vi "Simple.vi"() -> ()   [LabVIEW 2019]
doc: "A simple demonstration of encoding a cluster as MessagePack data and then decoding the MessagePack data back into the cluster. This shows how to use the high-level To Msgpack and From Msgpack VIs to convert anything into MessagePack data and convert MessagePack data based on a schema."
uses:
  vi.lib/Field R&D Services/LabPack/LabPack.lvlib
panel:
  in  "Input":cluster{"Compact":bool, "Schema":i32}={"Compact"=TRUE, "Schema"=0}
  out "Msgpack Data":string
  out "Output":cluster{"Compact":bool, "Schema":i32}
  # "Run the VI to see the input cluster encoded as MessagePack data and then decoded back to a cluster."
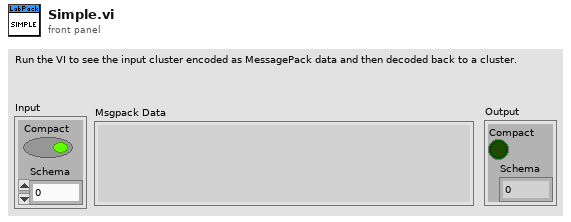
[diagram p1: front panel]
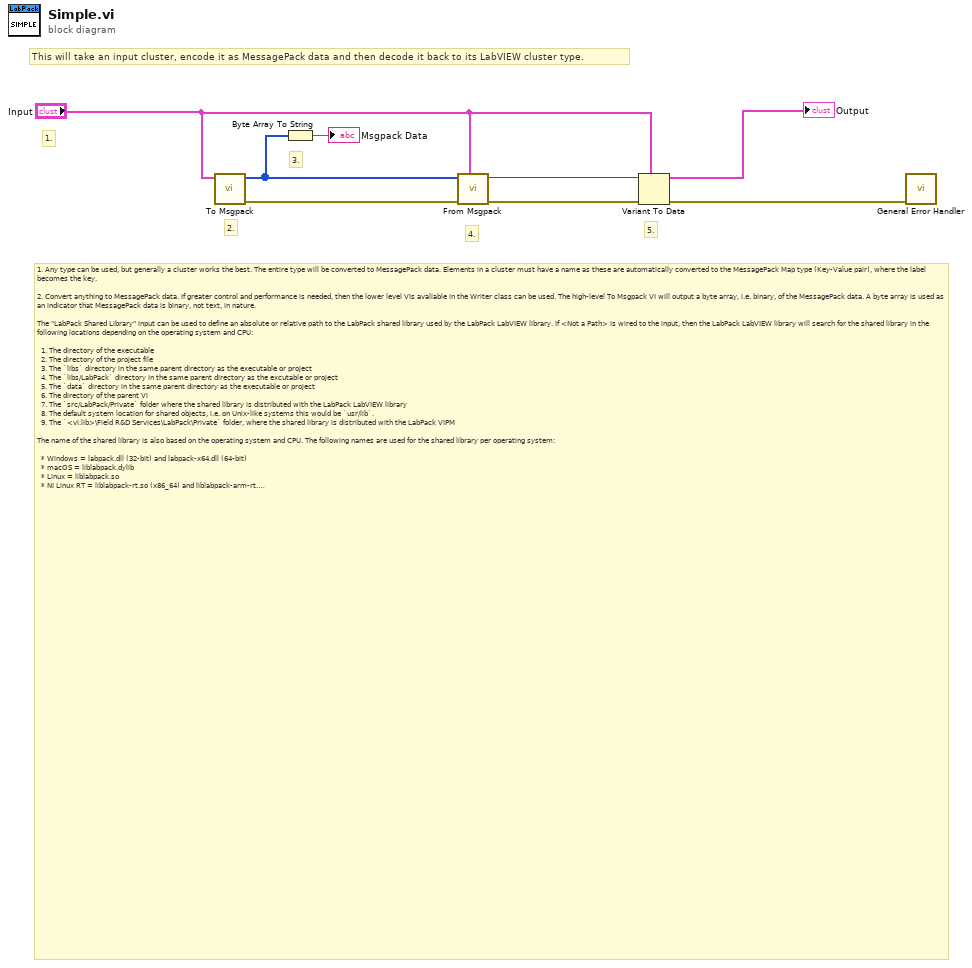
[diagram p0: block diagram]
diagram:
  # "1."
  # "This will take an input cluster, encode it as MessagePack data and then decode it back to its LabVIEW cluster type."
  # "1. Any type can be used, but generally a cluster works the best. The entire type will be converted to MessagePack data. Elements in a cluster must have a name as these are automatically converted to the MessagePack Map type (Key-Value pair), where the label becomes the key.\n\n2. Convert anything to MessagePack data. If greater control and performance is needed, then the lower level VIs avaliable in the Writer class can be used. The high-level To Msgpack VI will output a byte array, i.e. binary, of the MessagePack data. A byte array is used as an indicator that MessagePack data is binary, not text, in nature. \n\nThe \"LabPack Shared Library\" input can be used to define an absolute or relative path to the LabPack shared library used by the LabPack LabVIEW library. If <Not a Path> is wired to the input, then the LabPack LabVIEW library will search for the shared library in the following locations depending on the operating system and CPU: \n\n  1. The directory of the executable \n  2. The directory of the project file\n  3. The `libs` directory in the same parent directory as the executable or project\n  4. The `libs/LabPack` directory in the same parent directory as the excutable or project\n  5. The `data` directory in the same parent directory as the executable or project\n  6. The directory of the parent VI\n  7. The `src/LabPack/Private` folder where the shared library is distributed with the LabPack LabVIEW library\n  8. The default system location for shared objects, i.e. on Unix-like systems this would be `usr/lib`.\n  9. The `<vi.lib>\\Field R&D Services\\LabPack\\Private` folder, where the shared library is distributed with the LabPack VIPM\n\nThe name of the shared library is also based on the operating system and CPU. The following names are used for the shared library per operating system:\n\n  * Windows = labpack.dll (32-bit) and labpack-x64.dll (64-bit)\n  * macOS = liblabpack.dylib\n  * Linux = liblabpack.so\n  * NI Linux RT = liblabpack-rt.so (x86_64) and liblabpack-arm-rt.so (ARM)\n\nIf building a real-time application or executable with the Application Builder, the appropriate shared library must be installed on the target machine. For example, the liblabpack-rt.so must be transferred and \"installed\" on a NI Linux RT remote target in one of the locations listed above or in another location with a known path that can be passed to the \"LabPack Shared Library\" input.\n\n(i) Current Working Directory, (ii) the source (src) folder, and the system-specific shared library folder, i.e. \"/usr/lib/\" on Unix-like operating systems including Real-Time targets. The LabPack shared library must be present on disk. When creating an executable that uses the LabPack library, ensure the LabPack shared library is installed on the target in a known location and this path is used with the \"LabPack Shared Library\" input.\n\n3. Use the Byte Array to String primitive to make the MessagePack data more human-readable as a string in hex notation. Note, MessagePack data is binary and thus best viewed by a human in hex notation.\n\n4. Convert a byte array, i.e. binary data, in the MessagePack format to a LabVIEW type based on a \"schema\", which indicates the structure of the MessagePack data. Currently, the LabPack library does NOT support schema-less decoding of MessagePack data. If greater control and/or performance is needed, then the lower level VIs available in the Reader class can be used. The high-level From Msgpack VI is essentially a wrapper for the low-level Reader VIs. The \"LabPack Shared Library\" input can be used to define an absolute path to the LabPack shared library used by the LabPack LabVIEW library. If Not a Path is wired to the input, then the LabPack LabVIEW library will search for the shared library in the following locations: (i) Current Working Directory, (ii) the source (src) folder, and the system-specific shared library folder, i.e. \"/usr/lib/\" on Unix-like operating systems including Real-Time targets. The LabPack shared library must be present on disk. When creating an executable that uses the LabPack library, ensure the LabPack shared library is installed on the target in a known location and this path is used with the \"LabPack Shared Library\" input.\n\n5. Since any type can be used as a schema for decoding MessagePack data, a variant is used as the output of the From Msgpack VI. This variant must be converted to a LabVIEW type for further use."
  # "3."
  # "5."
  # "4."
  # "2."
  n1 = call "To Msgpack.vi"("Anything"="Input") -> ("Error Out"=w8:errorcluster, "Msgpack Data"=w2:u8[])  [unwired: 9 in]
  n2 = Byte Array To String(unsigned byte array=w2) -> (string=→"Msgpack Data":string)
  n3 = call "From Msgpack.vi"("Types and Defaults"="Input", "Error In"=w8, "Msgpack Data"=w2) -> ("Error Out"=w7:errorcluster, "Value"=w6:variant)  [unwired: 7 in]
  n4 = Variant To Data(error in=w7, type="Input", Variant=w6) -> (data=→"Output":cluster{"Compact":bool, "Schema":i32}, error out=w3:errorcluster)
  n5 = call <vilib>:"General Error Handler.vi"("error in (no error)"=w3) -> ()  [unwired: 10 in, 5 out]
